vi "Write Value.vi"(8 "error in (no error)":errorcluster, 10 "Value":dbl, 11 "Set Double Float in":refnum<class "Set Double Float.lvclass">) -> (0 "error out":errorcluster, 3 "Set Double Float out":refnum<class "Set Double Float.lvclass">)   [LabVIEW 2021, in "BT.lvlib" / "Set Double Float.lvclass"]
uses:
  Set Double Float.lvclass
  Set Double Float.lvclass/Set Double Float.ctl
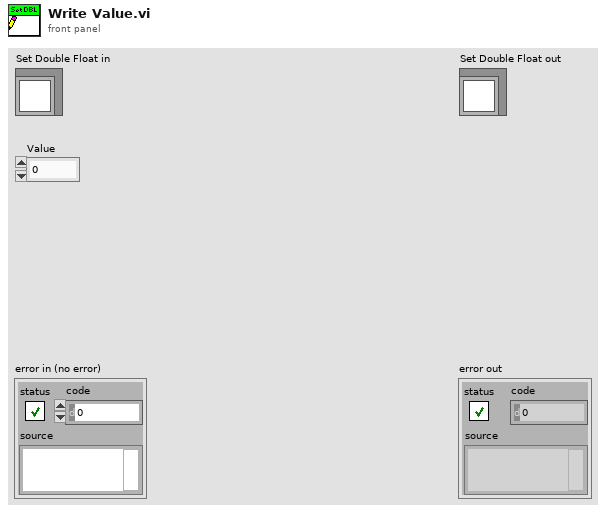
[diagram p1: front panel]
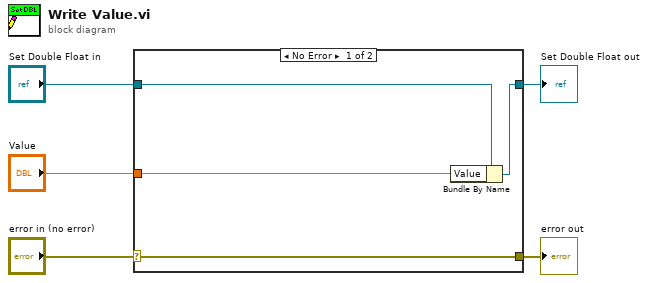
[diagram p0: block diagram]
diagram:
  n1 = case shown="No Error" "error in (no error)" {
    selector: "error in (no error)" -> [w9 w10]
    tunnel: [w9 w10] -> w4
    tunnel: [w7 w11] -> w2
    tunnel: "Set Double Float in" -> [w8 w11]
    tunnel: "Value" -> [w6 _]
    frame No Error {
      n2 = Bundle By Name(cluster=w8, "Value"=w6) -> (w7:refnum<class "Set Double Float.lvclass">)
    }
    frame Error {
    }
  }
  "error out" <- w4
  "Set Double Float out" <- w2
